vi "Create Lock String.vi"() -> (3 "String":string)   [LabVIEW 2016, in "Drive System.lvlib"]
uses:
  Drive System.lvlib
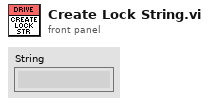
[diagram p1: front panel]
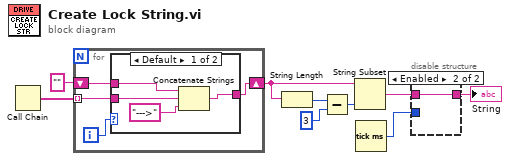
[diagram p0: block diagram]
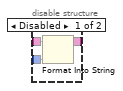
[diagram p2: hidden frame]
diagram:
  n1 = Call Chain() -> (call chain=w9:string[])
  n2 = for {
    tunnel: w9 -> [w12] mode=indexing
    shift-right: [w11] -> w7
    shift-left: "" -> [w10]
    i -> [w13]
    n3 = case shown="Default" w13 {
      tunnel: w12 -> [w17 _]
      tunnel: [w16 w18] -> w11
      tunnel: w10 -> [w15 w18]
      frame Default {
        n4 = Concatenate Strings(w15, w17, "--->" ("string")) -> (w16:string)
      }
      frame 0 {
      }
    }
  }
  n5 = String Length(string=w7) -> (length=w6:i32)
  n6 = Subtract(x=w6, y=3) -> (x-y=w4:i32)
  n7 = String Subset(string=w7, length (rest)=w4) -> (substring=w3:string)  [unwired: 1 in]
  n8 = Tick Count (ms)() -> (millisecond timer value=w1:u32)
  n9 = disable-structure shown="Enabled" {
    disable-tunnel: w3 -> [w21 w22]
    disable-tunnel: [w20 w22] -> w2
    disable-tunnel: w1 -> [w19 _]
    frame Disabled {
      n10 = Format Into String(initial string=w21, w19) -> (resulting string=w20:string)  [unwired: 2 in, 1 out]
    }
    frame Enabled {
    }
  }
  "String" <- w2
